vi "AddControlPanel.vi"(9 "Control panel done":bool, 10 "Control panel up":bool, 11 "Refnum in":T1) -> (3 "Refnum out":T1)   [LabVIEW 2019]
uses:
  <vilib>/vision/Image Controls.llb/IMAQ Image.ctl
  <vilib>/vision/NI_Vision_Development_Module.lvlib
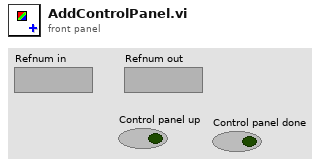
[diagram p1: front panel]
types:
  T1 = typedef "IMAQ Image.ctl" = refnum<image>
  T2 = typedef "Image Type" = u32
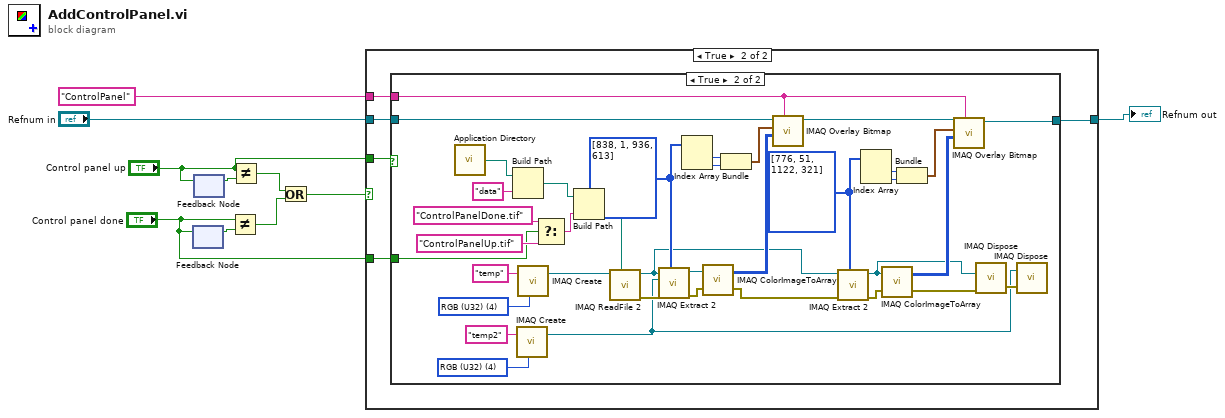
[diagram p0: block diagram]
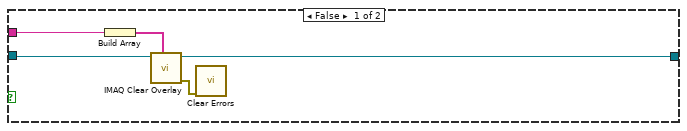
[diagram p3: hidden frame]
diagram:
  n1 = feedback #1() -> (w9:bool)  [unwired: 1 in]
  n2 = feedback-in #1("Control panel done") -> ()
  n3 = feedback #2() -> (w10:bool)  [unwired: 1 in]
  n4 = feedback-in #2("Control panel up") -> ()
  n5 = Not Equal?(x="Control panel done", y=w9) -> (x != y?=w8:bool)
  n6 = Not Equal?(x="Control panel up", y=w10) -> (x != y?=w3:bool)
  n7 = Or(x=w3, y=w8) -> (x .or. y?=w4:bool)
  n8 = case shown="True" w4 {
    tunnel: [w11 w15] -> w7
    tunnel: "Refnum in" -> [w11 w16]
    tunnel: "ControlPanel" -> [_ w14]
    tunnel: "Control panel up" -> [_ w13]
    tunnel: "Control panel done" -> [_ w12]
    frame False {
    }
    frame True {
      n9 = case shown="True" w13 {
        tunnel: w16 -> [w21 w58]
        tunnel: [w20 w38] -> w15
        tunnel: w14 -> [w19 w37]
        tunnel: w12 -> [_ w40]
        frame False {
          n10 = Build Array(w19) -> (w18:string[])
          n11 = call "IMAQ Clear Overlay"("Groups"=w18, "Image"=w21) -> ("error out"=w17:errorcluster, "Image Out"=w20:T1)  [unwired: 8 in]
          n12 = call <vilib>:"Clear Errors.vi"("error in (no error)"=w17) -> ()  [unwired: 5 in, 2 out]
        }
        frame True {
          w26 = T2 4 items=["Grayscale (U8)", "Grayscale (I16)", "Grayscale (SGL)", "Complex (CSG)", "RGB (U32)", "HSL (U32)", "RGB (U64)", "Grayscale (U16)"] ("Image Type")
          w27 = i32[] [776, 51, 1122, 321] ("Optional Rectangle")
          w47 = i32[] [838, 1, 936, 613] ("Optional Rectangle")
          w52 = T2 4 items=["Grayscale (U8)", "Grayscale (I16)", "Grayscale (SGL)", "Complex (CSG)", "RGB (U32)", "HSL (U32)", "RGB (U64)", "Grayscale (U16)"] ("Image Type")
          n13 = call <vilib>:"Application Directory.vi"() -> ("Application Directory"=w56:path)
          n14 = Build Path(base path=w56, name or relative path="data") -> (appended path=w57:path)
          n15 = call "IMAQ Create"("Image Name"="temp2", "Image Type"=w26) -> ("New Image"=w22:T1)  [unwired: 3 in, 1 out]
          n16 = call "IMAQ Create"("Image Name"="temp", "Image Type"=w52) -> ("New Image"=w51:T1)  [unwired: 3 in, 1 out]
          n17 = Select(t="ControlPanelDone.tif" ("name or relative path"), s=w40, f="ControlPanelUp.tif" ("name or relative path")) -> (s? t:f=w43:string)
          n18 = Build Path(base path=w57, name or relative path=w43) -> (appended path=w54:path)
          n19 = call "IMAQ ReadFile 2"("File Path"=w54, "Image"=w51) -> ("error out"=w50:errorcluster, "Image Out"=w24:T1)  [unwired: 5 in, 3 out]
          n20 = call "IMAQ Extract 2"("Optional Rectangle"=w47, "error in (no error)"=w50, "Image Dst"=w22, "Image Src"=w24) -> ("error out"=w49:errorcluster, "Image Dst Out"=w35:T1)  [unwired: 6 in]
          n21 = Index Array(array=w47) -> (element #1=w45:i32, element #2=w46:i32)  [unwired: 2 in]
          n22 = call "IMAQ ColorImageToArray"("Image"=w35, "error in (no error)"=w49) -> ("Image Pixels (U32)"=w48:u32[][], "error out"=w33:errorcluster)  [unwired: 2 in, 1 out]
          n23 = Bundle(w45, w46) -> (w44:cluster{i32, i32})  [unwired: 1 in]
          n24 = call "IMAQ Overlay Bitmap"("Group"=w37, "Bitmap"=w48, "Top Left Point"=w44, "Image"=w58) -> ("Image Out"=w39:T1)  [unwired: 6 in, 1 out]
          n25 = call "IMAQ Extract 2"("Optional Rectangle"=w27, "error in (no error)"=w33, "Image Src"=w24) -> ("error out"=w36:errorcluster, "Image Dst Out"=w31:T1)  [unwired: 7 in]
          n26 = Index Array(array=w27) -> (element #1=w30:i32, element #2=w29:i32)  [unwired: 2 in]
          n27 = call "IMAQ ColorImageToArray"("Image"=w31, "error in (no error)"=w36) -> ("Image Pixels (U32)"=w34:u32[][], "error out"=w32:errorcluster)  [unwired: 2 in, 1 out]
          n28 = Bundle(w30, w29) -> (w28:cluster{i32, i32})  [unwired: 1 in]
          n29 = call "IMAQ Overlay Bitmap"("Group"=w37, "Bitmap"=w34, "Top Left Point"=w28, "Image"=w39) -> ("Image Out"=w38:T1)  [unwired: 6 in, 1 out]
          n30 = call "IMAQ Dispose"("Image"=w31, "error in (no error)"=w32) -> ("error out"=w23:errorcluster)  [unwired: 4 in]
          n31 = call "IMAQ Dispose"("Image"=w22, "error in (no error)"=w23) -> ()  [unwired: 4 in, 1 out]
        }
      }
    }
  }
  "Refnum out" <- w7
